vi "Set Perimiters.vi"(11 "Plant Regions":map{T1, u32}[](array[numeric])) -> (3 "Plant Regions 2":map{T1, u32}[](array[numeric]))   [LabVIEW 2024]
uses:
  Utility/Universal Utility/TypeDefs_Utility/Cluster_Row-Column.ctl
  Utility/Universal Utility/TypeDefs_Utility/ENUM_4 Directions U-D-L-R.ctl
  <vilib>/Utility/miscctls.llb/LVMapReplaceAction.ctl
  9ec40043-fd1c-4aa8-aa2f-c598280360ae.vi
  9ec40043-fd1c-4aa8-aa2f-c598280360ae.vi/0a5f5d0f-6921-449f-9499-5f6c7f3eae0e.vi
  9ec40043-fd1c-4aa8-aa2f-c598280360ae.vi/2f57c213-34d0-4fb8-93c4-9da21d141025.vi
  <vilib>/Utility/error.llb/Trim Whitespace.vi
  <vilib>/Utility/error.llb/Trim Whitespace One-Sided.vi
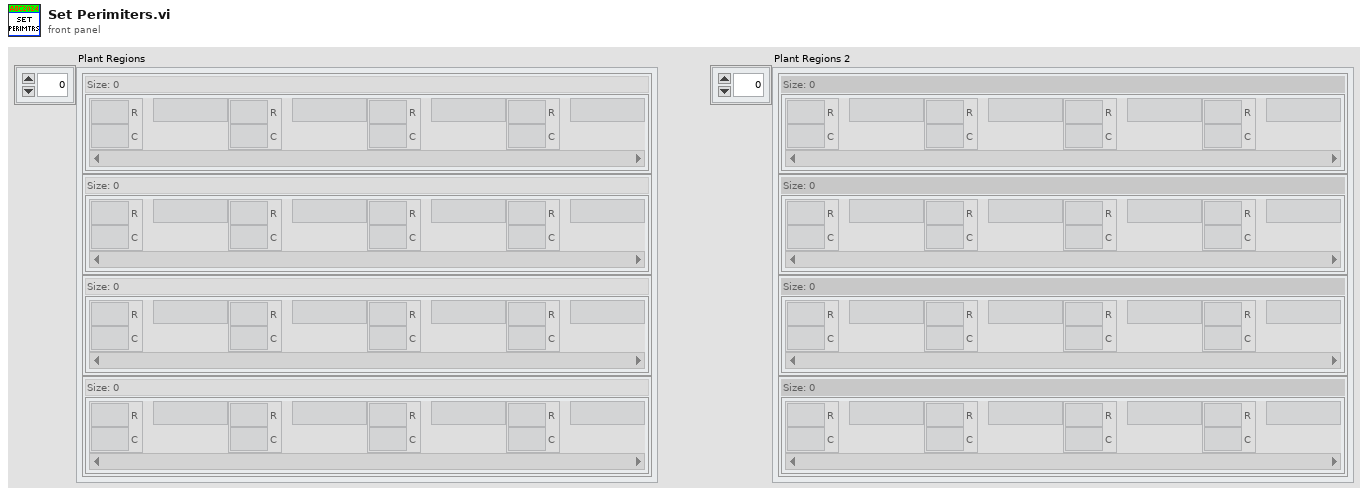
[diagram p1: front panel]
types:
  T1 = typedef "Cluster_Row-Column.ctl" = cluster{"R":i32, "C":i32}
  T2 = typedef "ENUM_4 Directions U-D-L-R.ctl" = enum16{"Up;-1,0", "Right;0,1", "Down;1,0", "Left;0,-1"}
  T3 = typedef "LVMapReplaceAction.ctl" = enum32{"Modify Entry only if found", "Add or Modify Entry", "Delete Entry"}
  T4 = typedef "Cluster_X-Y.ctl" = cluster{"X":u64, "Y":u64}
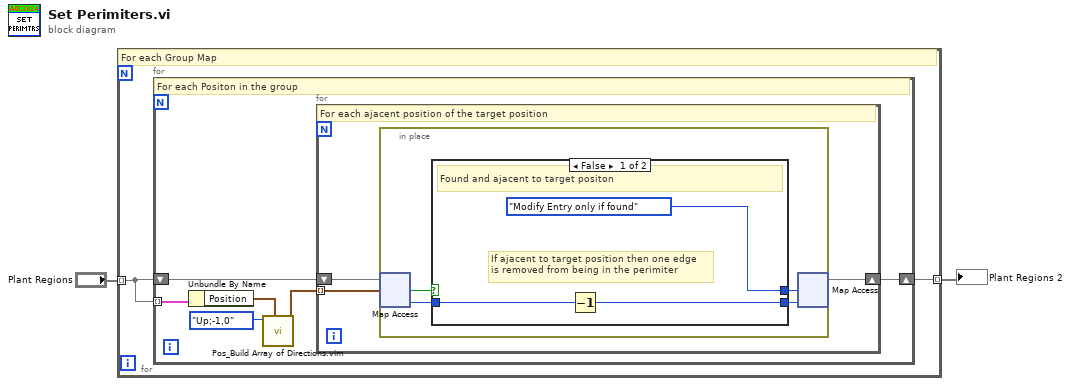
[diagram p0: block diagram]
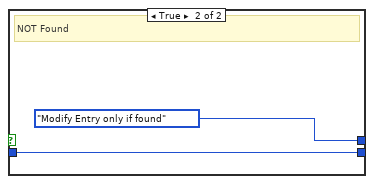
[diagram p2: hidden frame]
diagram:
  n1 = for {
    tunnel: "Plant Regions" -> [w4] mode=indexing
    tunnel: [w3] -> w1 mode=indexing
    # "For each Group Map"
    n2 = for {
      tunnel: w4 -> [w10] mode=indexing
      shift-right: [w7] -> w3
      shift-left: w4 -> [w8]
      # "For each Positon in the group"
      n3 = Unbundle By Name(w10) -> ("Position"=w5:T1)
      n4 = call "Pos_Build Array of Directions.vim"("Positon"=w5, "Direction"=ENUM_4_Directions_U-D-L-R."Up;-1,0") -> ("Direction Positions Out"=w6:T4[])  [unwired: 9 in]
      n5 = for {
        tunnel: w6 -> [w11] mode=indexing
        shift-right: [w12] -> w7
        shift-left: w8 -> [w13]
        # "For each ajacent position of the target position"
        n6 = in-place {
          n7 = in-place-map #1(w13, w11) -> (w17:u32, w15:bool)  [unwired: 1 in]
          n8 = case shown="False" w15 {
            tunnel: w17 -> [w19 w21]
            tunnel: [LVMapReplaceAction."Modify Entry only if found" ("action") LVMapReplaceAction."Modify Entry only if found" ("action")] -> w16
            tunnel: [w18 w21] -> w14
            frame False {
              # "If ajacent to target position then one edge\nis removed from being in the perimiter"
              # "Found and ajacent to target positon"
              n9 = Decrement(x=w19) -> (x-1=w18:u32)
            }
            frame True {
              # "NOT Found"
            }
          }
          n10 = in-place-map #1(w14, w16) -> (w12:map{T1, u32})  [unwired: 2 out]
        }
      }
    }
  }
  "Plant Regions 2" <- w1
